vi "Control to String.vi"(8 "error in (no error)":errorcluster, 11 "Limit":refnum<vi>) -> (0 "error out":errorcluster, 2 "error":bool, 3 "StringLimit":string[](array[string]))   [LabVIEW 2019, in "TestSetup.lvlib" / "TestSetup.lvclass"]
uses:
  TestSetup.lvclass
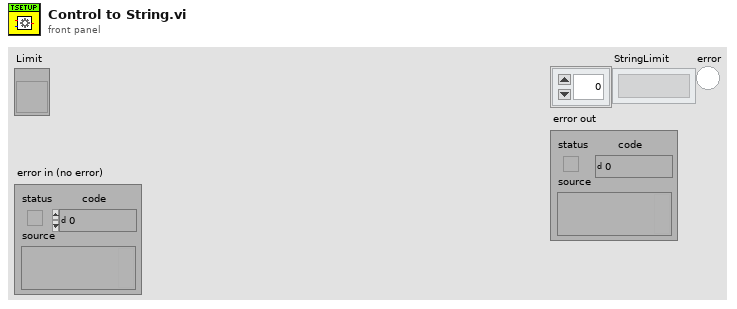
[diagram p1: front panel]
types:
  T1 = typedef "TestSetup.lvlib/TestSetup.lvclass/Limit.ctl" = cluster{"ItemName":string, "Type":enum16{"I8", "I16", "I32", "I64", "U8", "U16", "U32", "U64", "Double Float", "Boolean", "String", "Numeric Array", "String Array"}, "LowLimit":string, "HighLimit":string}
  T2 = enum16{"I8", "I16", "I32", "I64", "U8", "U16", "U32", "U64", "Double Float", "Boolean", "String", "Numeric Array", "String Array"}
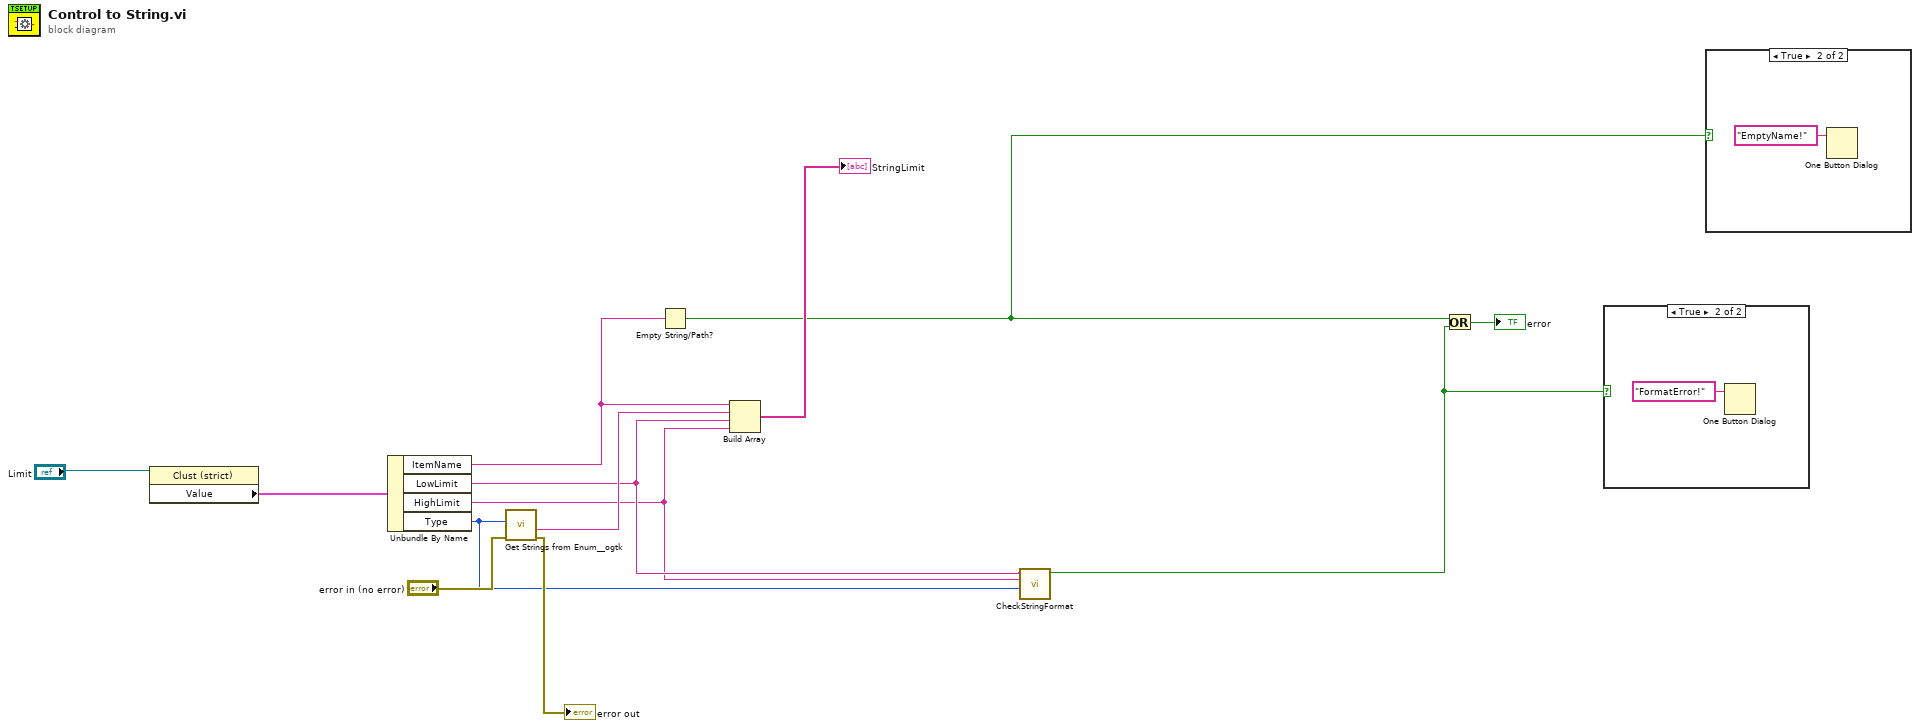
[diagram p0: block diagram]
diagram:
  n1 = property class="Clust (strict)"(reference="Limit") -> ("Value"=w13:T1)  [unwired: 1 in, 2 out]
  n2 = Unbundle By Name(w13) -> ("ItemName"=w11:string, "LowLimit"=w6:string, "HighLimit"=w5:string, "Type"=w4:T2)
  n3 = call <userlib>:"Get Strings from Enum__ogtk.vi"("error in (no error)"="error in (no error)", "Enum"=w4) -> ("error out"=→"error out":errorcluster, "String Value"=w9:string)  [unwired: 6 in, 2 out]
  n4 = Empty String/Path?(string/path=w11) -> (empty?=w3:bool)
  n5 = Build Array(w11, w9, w6, w5) -> (→"StringLimit":string[])
  n6 = call "CheckStringFormat.vi"("Type"=w4, "HighLimit"=w5, "LowLimit"=w6) -> ("status"=w2:bool)  [unwired: 8 in]
  n7 = Or(x=w3, y=w2) -> (x .or. y?=→"error":bool)
  n8 = case shown="True" w2 {
    frame False {
    }
    frame True {
      n9 = One Button Dialog(message="FormatError!") -> ()  [unwired: 1 in, 1 out]
    }
  }
  n10 = case shown="True" w3 {
    frame False {
    }
    frame True {
      n11 = One Button Dialog(message="EmptyName!") -> ()  [unwired: 1 in, 1 out]
    }
  }
